vi "DAQ AO.vi"(7 "Signals":T6, 10 "Action":T5, 11 "Params":T4) -> (9 "Status":T3)   [LabVIEW 2020, in "DAQmx AO.lvlib"]
uses:
  DAQmx AO.lvlib
  <extravilib>/ChannelInstances/Flex-t'DAQmx AO.lvlib-Action.ctl'.lvlib
  <extravilib>/ChannelInstances/Flex-t'DAQmx AO.lvlib-Params.ctl'.lvlib
  Params.ctl
  <extravilib>/ChannelInstances/Flex-t'DAQmx AO.lvlib-Params.ctl'/Event Data.ctl
  Action.ctl
  <extravilib>/ChannelInstances/Flex-t'DAQmx AO.lvlib-Action.ctl'/Event Data.ctl
  Write Event Data.ctl
  Status.ctl
  <extravilib>/ChannelInstances/Flex-t'DAQmx AO.lvlib-Status.ctl'.lvlib
  <vilib>/DAQmx/create/channels.llb/DAQmx Create Channel (AO-Voltage-Basic).vi
  <vilib>/DAQmx/configure/timing.llb/DAQmx Timing (Sample Clock).vi
  <extravilib>/ChannelInstances/Flex-a[.](wfm(dbl)).lvlib
  <vilib>/DAQmx/write.llb/DAQmx Write (Analog 1D Wfm NChan NSamp).vi
  <extravilib>/ChannelInstances/Flex-a[.](wfm(dbl))/))Channel.ctl
  <extravilib>/ChannelInstances/Flex-t'DAQmx AO.lvlib-Action.ctl'/))Channel.ctl
  <extravilib>/ChannelInstances/Flex-t'DAQmx AO.lvlib-Params.ctl'/))Channel.ctl
  <extravilib>/ChannelInstances/Flex-t'DAQmx AO.lvlib-Status.ctl'/))Channel.ctl
panel:
  out "Queued Count":i32[](array[numeric])
  out "Rate":dbl
  out "Graph":waveform(dbl)[](graph)
  out "error out":errorcluster
  out "task out":refnum<k21>
  out "Task Status":T1
  out "Task Params":T2 {"Sample Rate" format="%.3p"}
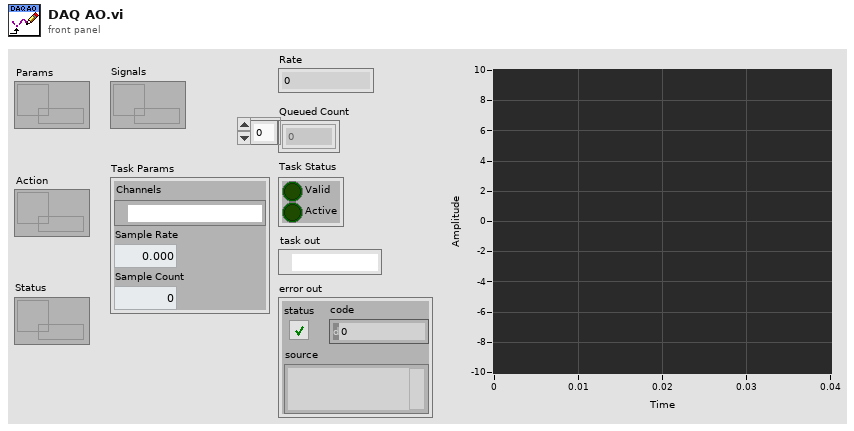
[diagram p1: front panel]
types:
  T1 = typedef "DAQmx AO.lvlib/Status.ctl" = cluster{"Valid":bool, "Active":bool}
  T2 = typedef "DAQmx AO.lvlib/Params.ctl" = cluster{"Channels":tag, "Sample Rate":dbl, "Sample Count":i32}
  T3 = typedef "Flex-t'DAQmx AO.lvlib-Status.ctl'.lvlib/))Channel.ctl" = refnum<queue>
  T4 = typedef "Flex-t'DAQmx AO.lvlib-Params.ctl'.lvlib/))Channel.ctl" = refnum<queue>
  T5 = typedef "Flex-t'DAQmx AO.lvlib-Action.ctl'.lvlib/))Channel.ctl" = refnum<queue>
  T6 = typedef "Flex-a[.](wfm(dbl)).lvlib/))Channel.ctl" = refnum<queue>
  T7 = typedef "DAQmx AO.lvlib/Write Event Data.ctl" = cluster{"Start":bool, "Stop":bool, "Close":bool}
  T8 = cluster{"Action":refnum<event-registration>, "Params":refnum<event-registration>, "Write":refnum<event-registration>}
  T9 = typedef "DAQmx AO.lvlib/Action.ctl" = enum16{"Verify", "Start", "Stop", "Close", "Error"}
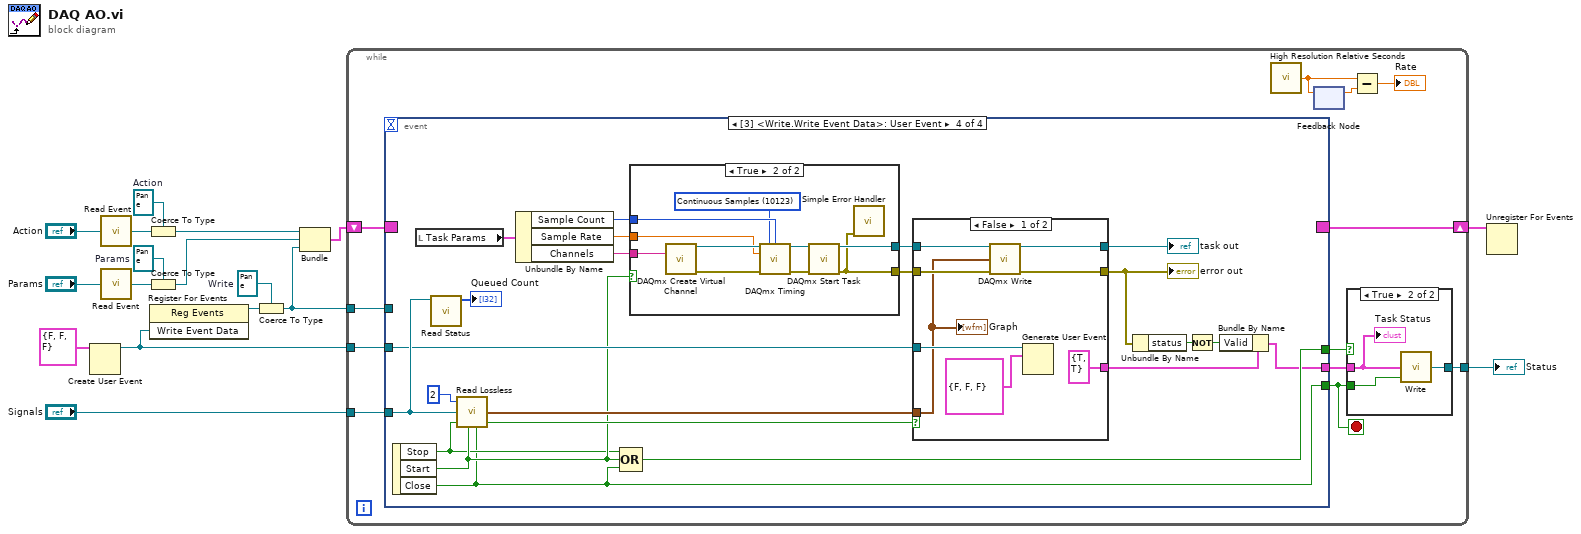
[diagram p0: block diagram]
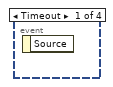
[diagram p3: hidden frame]
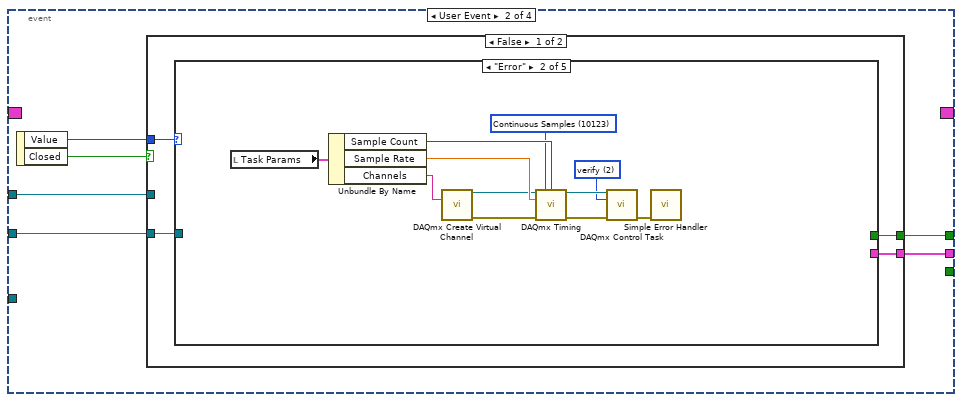
[diagram p4: hidden frame]
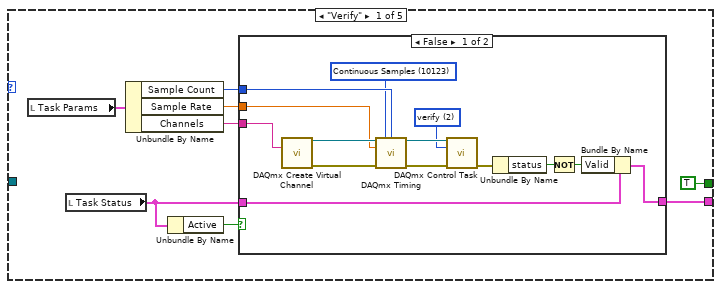
[diagram p5: hidden frame]
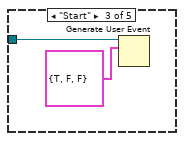
[diagram p7: hidden frame]
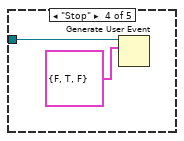
[diagram p8: hidden frame]
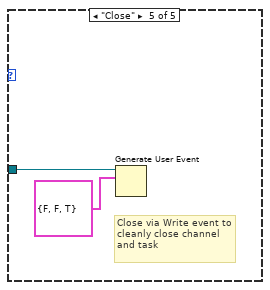
[diagram p9: hidden frame]
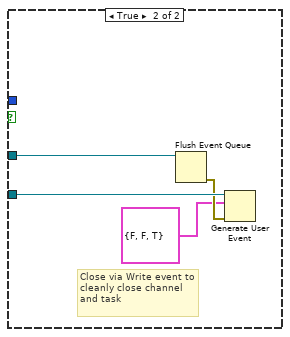
[diagram p10: hidden frame]
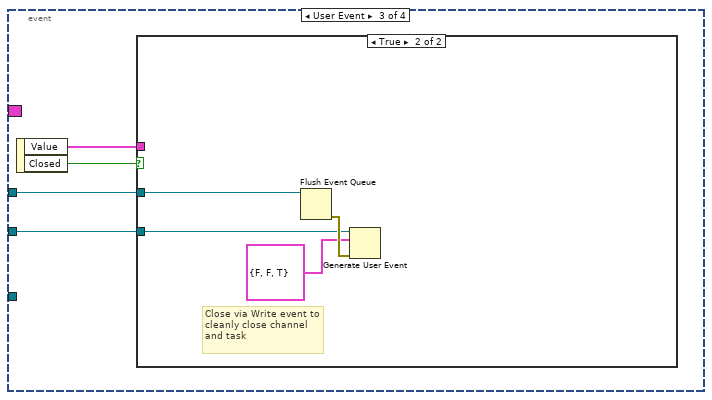
[diagram p11: hidden frame]
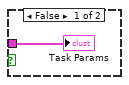
[diagram p12: hidden frame]
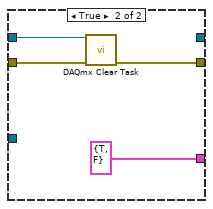
[diagram p13: hidden frame]
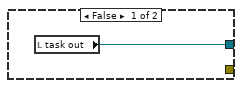
[diagram p14: hidden frame]
diagram:
  w4 = refnum<event-registration> refnum  # Write
  w10 = refnum<event-registration> refnum  # Action
  w13 = refnum<event-registration> refnum  # Params
  n1 = Create User Event(user event datatype=T7 {"Start"=FALSE, "Stop"=FALSE, "Close"=FALSE} ("Write Event Data")) -> (user event=w3:refnum<user-event>)  [unwired: 1 in, 1 out]
  n2 = call <extravilib>:"Read Event.vi"("FlexChannel"="Action") -> ("Event Reg"=w12:refnum<event-registration>)  [unwired: 8 in]
  n3 = call <extravilib>:"Read Event.vi"("FlexChannel"="Params") -> ("Event Reg"=w15:refnum<event-registration>)  [unwired: 8 in]
  n4 = Coerce To Type(0:w12, 1:w10) -> (2:w11:refnum<event-registration>)
  n5 = Coerce To Type(0:w15, 1:w13) -> (2:w14:refnum<event-registration>)
  n6 = register-events(w3) -> (reference out=w6:refnum<event-registration>)  [unwired: 2 in, 1 out]
  n7 = Coerce To Type(0:w6, 1:w4) -> (2:w2:refnum<event-registration>)
  n8 = Bundle("Action"=w11, "Params"=w14, "Write"=w2) -> (w9:T8)  [unwired: 1 in]
  n9 = while {
    shift-right: [w28] -> w8
    shift-left: w9 -> [w29]
    tunnel: "Signals" -> [w27]
    tunnel: w3 -> [w26]
    tunnel: w2 -> [w25]
    tunnel: [w24] -> w1
    stop <- w21 stop-if-true
    n10 = event shown="[3] <Write.Write Event Data>: User Event" {
      selector: w29 -> [_ _ _ _]
      dyn-events: [_ _ _ _] -> w28
      timeout: _ -> [_ _ _ _]
      tunnel: w27 -> [_ _ _ w113]
      tunnel: w26 -> [_ w36 w87 w107]
      tunnel: w25 -> [_ w35 w88 _]
      tunnel: [_ w34 _ w100] -> w23
      tunnel: [_ w33 _ w104] -> w22
      tunnel: [_ _ _ w99] -> w21
      event Timeout {
        n11 = event-data() -> ()  [unwired: 1 in, 1 out]
      }
      event User Event {
        n12 = event-data() -> ("Value"=w37:T9, "Closed"=w38:bool)  [unwired: 1 in]
        n13 = case shown="False" w38 {
          tunnel: w37 -> [w42 _]
          tunnel: w36 -> [w39 w85]
          tunnel: w35 -> [_ w86]
          tunnel: [w41 _] -> w34
          tunnel: [w40 _] -> w33
          frame False {
            n14 = case shown="\"Error\"" w42 {
              tunnel: [w46 _ _ _ _] -> w41
              tunnel: [TRUE _ _ _ _] -> w40
              tunnel: w39 -> [_ _ w77 w79 w82]
              frame "Verify" {
                n15 = local read "Task Params"() -> (w50:T2)
                n16 = local read "Task Status"() -> (w44:T1)
                n17 = Unbundle By Name(w50) -> ("Sample Count"=w48:i32, "Sample Rate"=w47:dbl, "Channels"=w49:tag)
                n18 = Unbundle By Name(w44) -> ("Active"=w43:bool)
                n19 = case shown="False" w43 {
                  tunnel: w49 -> [w64 _]
                  tunnel: w48 -> [w61 _]
                  tunnel: w47 -> [w59 _]
                  tunnel: [w52 w65] -> w46
                  tunnel: w44 -> [w51 w65]
                  frame False {
                    w57 = 2 items=["verify"=2, "reserve"=4, "commit"=3, "unreserve"=5, "abort"=6] ("action")
                    w60 = 10123 items=["Finite Samples"=10178, "Continuous Samples"=10123, "Hardware Timed Single Point"=12522] ("sample mode")
                    n20 = call-poly <vilib>:"DAQmx Create Virtual Channel.vi"("physical channels"=w64) -> ("task out"=w63:refnum<k21>, "error out"=w62:errorcluster)  [unwired: 13 in]
                    n21 = call-poly <vilib>:"DAQmx Timing.vi"("task/channels in"=w63, "sample mode"=w60, "samples per channel"=w61, "rate"=w59, "error in"=w62) -> ("task out"=w58:refnum<k21>, "error out"=w56:errorcluster)  [unwired: 9 in]
                    n22 = call <vilib>:"DAQmx Control Task.vi"("task/channels in"=w58, "action"=w57, "error in"=w56) -> ("error out"=w55:errorcluster)  [unwired: 11 in, 1 out]
                    n23 = Unbundle By Name(w55) -> ("status"=w54:bool)
                    n24 = Not(x=w54) -> (.not. x?=w53:bool)
                    n25 = Bundle By Name(cluster=w51, "Valid"=w53) -> (w52:T1)
                  }
                  frame True {
                  }
                }
              }
              frame "Error" {
                w68 = 2 items=["verify"=2, "reserve"=4, "commit"=3, "unreserve"=5, "abort"=6] ("action")
                w70 = 10123 items=["Finite Samples"=10178, "Continuous Samples"=10123, "Hardware Timed Single Point"=12522] ("sample mode")
                n26 = local read "Task Params"() -> (w76:T2)
                n27 = Unbundle By Name(w76) -> ("Sample Count"=w74:i32, "Sample Rate"=w73:dbl, "Channels"=w75:tag)
                n28 = call-poly <vilib>:"DAQmx Create Virtual Channel.vi"("physical channels"=w75) -> ("task out"=w72:refnum<k21>, "error out"=w71:errorcluster)  [unwired: 13 in]
                n29 = call-poly <vilib>:"DAQmx Timing.vi"("task/channels in"=w72, "sample mode"=w70, "samples per channel"=w74, "rate"=w73, "error in"=w71) -> ("task out"=w69:refnum<k21>, "error out"=w67:errorcluster)  [unwired: 9 in]
                n30 = call <vilib>:"DAQmx Control Task.vi"("task/channels in"=w69, "action"=w68, "error in"=w67) -> ("error out"=w66:errorcluster)  [unwired: 11 in, 1 out]
                n31 = call <vilib>:"Simple Error Handler.vi"("error in (no error)"=w66) -> ()  [unwired: 4 in, 5 out]
              }
              frame "Start" {
                n32 = Generate User Event(user event=w77, event data cluster=T7 {"Start"=TRUE, "Stop"=FALSE, "Close"=FALSE} ("event data")) -> ()  [unwired: 2 in, 2 out]
              }
              frame "Stop" {
                n33 = Generate User Event(user event=w79, event data cluster=T7 {"Start"=FALSE, "Stop"=TRUE, "Close"=FALSE} ("event data")) -> ()  [unwired: 2 in, 2 out]
              }
              frame "Close" {
                # "Close via Write event to cleanly close channel and task"
                n34 = Generate User Event(user event=w82, event data cluster=T7 {"Start"=FALSE, "Stop"=FALSE, "Close"=TRUE} ("event data")) -> ()  [unwired: 2 in, 2 out]
              }
            }
          }
          frame True {
            # "Close via Write event to cleanly close channel and task"
            n35 = Flush Event Queue(0:w86) -> (11:w84:errorcluster)  [unwired: 5 in, 2 out]
            n36 = Generate User Event(user event=w85, event data cluster=T7 {"Start"=FALSE, "Stop"=FALSE, "Close"=TRUE} ("event data"), error in=w84) -> ()  [unwired: 1 in, 2 out]
          }
        }
      }
      event User Event {
        n37 = event-data() -> ("Value"=w89:T2, "Closed"=w90:bool)  [unwired: 1 in]
        n38 = case shown="True" w90 {
          tunnel: w89 -> [w91 _]
          tunnel: w88 -> [_ w93]
          tunnel: w87 -> [_ w92]
          frame False {
            "Task Params" <- w91
          }
          frame True {
            # "Close via Write event to cleanly close channel and task"
            n39 = Flush Event Queue(0:w93) -> (11:w95:errorcluster)  [unwired: 5 in, 2 out]
            n40 = Generate User Event(user event=w92, event data cluster=T7 {"Start"=FALSE, "Stop"=FALSE, "Close"=TRUE} ("event data"), error in=w95) -> ()  [unwired: 1 in, 2 out]
          }
        }
      }
      event User Event {
        n41 = event-data() -> ("Stop"=w102:bool, "Start"=w103:bool, "Close"=w99:bool)  [unwired: 1 in]
        n42 = local read "Task Params"() -> (w117:T2)
        n43 = call <extravilib>:"Read Status.vi"("channel"=w113) -> ("Queued Count"=→"Queued Count":i32[])  [unwired: 4 in, 6 out]
        n44 = call <extravilib>:"Read Lossless.vi"("Depth (Unlimited)"=2, "FlexChannel"=w113, "Release (F)"=w102, "Restart (F)"=w103, "Close All (F)"=w99) -> ("Element"=w111:waveform(dbl)[], "Closed?"=w110:bool)  [unwired: 1 in, 2 out]
        n45 = Unbundle By Name(w117) -> ("Sample Count"=w116:i32, "Sample Rate"=w115:dbl, "Channels"=w114:tag)
        n46 = Compound Arithmetic op=OR(w102, w103, w99) -> (w104:bool)
        n47 = case shown="True" w103 {
          tunnel: w116 -> [_ w138]
          tunnel: w115 -> [_ w137]
          tunnel: w114 -> [_ w136]
          tunnel: [w130 w132] -> w109
          tunnel: [_ w131] -> w108
          frame False {
            n48 = local read "task out"() -> (w130:refnum<k21>)
          }
          frame True {
            w135 = 10123 items=["Finite Samples"=10178, "Continuous Samples"=10123, "Hardware Timed Single Point"=12522] ("sample mode")
            n49 = call-poly <vilib>:"DAQmx Create Virtual Channel.vi"("physical channels"=w136) -> ("task out"=w140:refnum<k21>, "error out"=w139:errorcluster)  [unwired: 13 in]
            n50 = call-poly <vilib>:"DAQmx Timing.vi"("task/channels in"=w140, "sample mode"=w135, "samples per channel"=w138, "rate"=w137, "error in"=w139) -> ("task out"=w134:refnum<k21>, "error out"=w133:errorcluster)  [unwired: 9 in]
            n51 = call <vilib>:"DAQmx Start Task.vi"("task/channels in"=w134, "error in"=w133) -> ("task out"=w132:refnum<k21>, "error out"=w131:errorcluster)  [unwired: 12 in]
            n52 = call <vilib>:"Simple Error Handler.vi"("error in (no error)"=w131) -> ()  [unwired: 4 in, 5 out]
          }
        }
        n53 = case shown="False" w110 {
          tunnel: w111 -> [w118 _]
          tunnel: w109 -> [w125 w129]
          tunnel: w108 -> [w124 w128]
          tunnel: w107 -> [w123 _]
          tunnel: [w122 _] -> w106
          tunnel: [w121 w127] -> w98
          tunnel: [T1 {"Valid"=TRUE, "Active"=TRUE} ("Task Status") T1 {"Valid"=TRUE, "Active"=FALSE} ("Task Status")] -> w101
          frame False {
            n54 = call-poly <vilib>:"DAQmx Write.vi"("task/channels in"=w125, "data"=w118, "error in"=w124) -> ("task out"=w122:refnum<k21>, "error out"=w121:errorcluster)  [unwired: 10 in, 1 out]
            n55 = Generate User Event(user event=w123, event data cluster=T7 {"Start"=FALSE, "Stop"=FALSE, "Close"=FALSE} ("event data")) -> ()  [unwired: 2 in, 2 out]
            "Graph" <- w118
          }
          frame True {
            n56 = call <vilib>:"DAQmx Clear Task.vi"("task in"=w129, "error in"=w128) -> ("error out"=w127:errorcluster)  [unwired: 13 in]
          }
        }
        "task out" <- w106
        "error out" <- w98
        n57 = Unbundle By Name(w98) -> ("status"=w97:bool)
        n58 = Not(x=w97) -> (.not. x?=w96:bool)
        n59 = Bundle By Name(cluster=w101, "Valid"=w96) -> (w100:T1)
      }
    }
    n60 = call <vilib>:"High Resolution Relative Seconds.vi"() -> ("relative seconds"=w19:dbl)
    n61 = feedback-in #1(w19) -> ()
    n62 = feedback #1() -> (w20:dbl)  [unwired: 1 in]
    n63 = case shown="True" w22 {
      tunnel: [_ w32] -> w24
      tunnel: w23 -> [_ w31]
      tunnel: w21 -> [_ w30]
      frame False {
      }
      frame True {
        n64 = call <extravilib>:"Write.vi"("element"=w31, "Close? (F)"=w30) -> ("channel"=w32:T3)  [unwired: 5 in, 2 out]
        "Task Status" <- w31
      }
    }
    n65 = Subtract(x=w19, y=w20) -> (x-y=→"Rate":dbl)
  }
  "Status" <- w1
  n66 = Unregister For Events(event registration refnum=w8) -> ()  [unwired: 1 in, 1 out]
